vi "Firmware_Update Dialog.vi"() -> ()   [LabVIEW 2011, in "CAN FD.lvlib"]
uses:
  CAN FD.lvlib
panel:
  in  "Cancel":bool
  in  "OK":bool
  in  "Pwd":string caption="密码"
  # "说明：点击确认后，PC会出现一个U盘，进入到U盘，将里\n面的firmware.bin文件删除，然后将新的firmware.bin文件\n存入其中，确保成功后，方可重新拔插USB线。"
  # "注意：请确保文件已经存入U盘，否则会导致刷新失\n败，无法运行。"
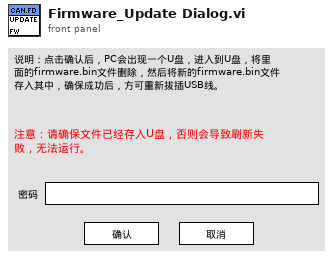
[diagram p1: front panel]
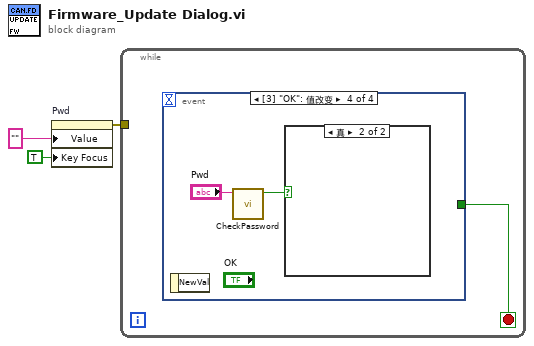
[diagram p0: block diagram]
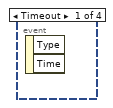
[diagram p2: hidden frame]
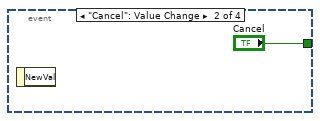
[diagram p3: hidden frame]
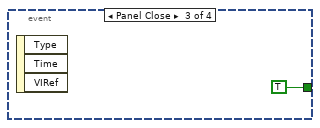
[diagram p4: hidden frame]
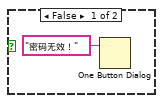
[diagram p5: hidden frame]
diagram:
  n1 = property on="Pwd" class="Str"("Value"="" ("Pwd"), "Key Focus"=TRUE ("键选中")) -> (error out=w1:errorcluster)  [unwired: 2 in, 1 out]
  n2 = while {
    tunnel: w1 -> [_]
    stop <- w4 stop-if-true
    n3 = event shown="[3] \"OK\": 值改变" {
      selector: _ -> [_ _ _ _]
      dyn-events: _ -> [_ _ _ _]
      timeout: _ -> [_ _ _ _]
      tunnel: [_ "Cancel" TRUE ("Cancel") _] -> w4
      event Timeout {
        n4 = event-data() -> ()  [unwired: 1 in, 2 out]
      }
      event "Cancel": Value Change {
        n5 = event-data() -> ()  [unwired: 1 in, 1 out]
      }
      event Panel Close {
        n6 = event-data() -> ()  [unwired: 1 in, 3 out]
      }
      event "OK": Value Change {
        n7 = event-data() -> ()  [unwired: 1 in, 1 out]
        n8 = call "CheckPassword.vi"("Password"="Pwd") -> ("Pass?"=w7:bool)  [unwired: 10 in]
        n9 = case shown="真" w7 {
          frame False {
            n10 = One Button Dialog(message="密码无效！" ("消息")) -> ()  [unwired: 1 in, 1 out]
          }
          frame True {
          }
        }
      }
    }
  }
